vi "Write.vi"(10 "String Array":string[](array[string]), 11 "String Array in":refnum<class "String Array.lvclass">) -> (3 "String Array out":refnum<class "String Array.lvclass">)   [LabVIEW 2020, in "Data.lvlib" / "String Array.lvclass"]
doc: "Write String Array."
uses:
  String Array.lvclass
  String Array.lvclass/String Array.ctl
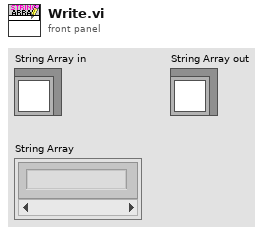
[diagram p1: front panel]
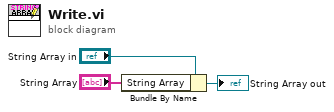
[diagram p0: block diagram]
diagram:
  n1 = Bundle By Name(cluster="String Array in", "String Array"="String Array") -> (→"String Array out":refnum<class "String Array.lvclass">)
